vi "动力和环境监控系统首页.vi"() -> ()   [LabVIEW 2016, in "环境动力监测库.lvlib"]
panel:
  out "网络状态":bool
  out "安防模块":T1
  out "暖通模块":T2
  out "供电模块":T3 {"蓄电池"."电量" format="%.0f %"; "蓄电池"."电池电量:" scale=0.0..100.0; "UPS"."电量" format="%.0f %"; "UPS"."电池电量:" scale=0.0..100.0}
  # "安防模块"
  # "供电模块"
  # "其他"
  # "暖通模块"
  # "真角"
  # "m/s"
  # "℃"
  # "bars"
  # "℃"
  # "℃"
  # "℃"
  # "V"
  # "V"
  # "V"
  # "V"
  # "V"
  # "A"
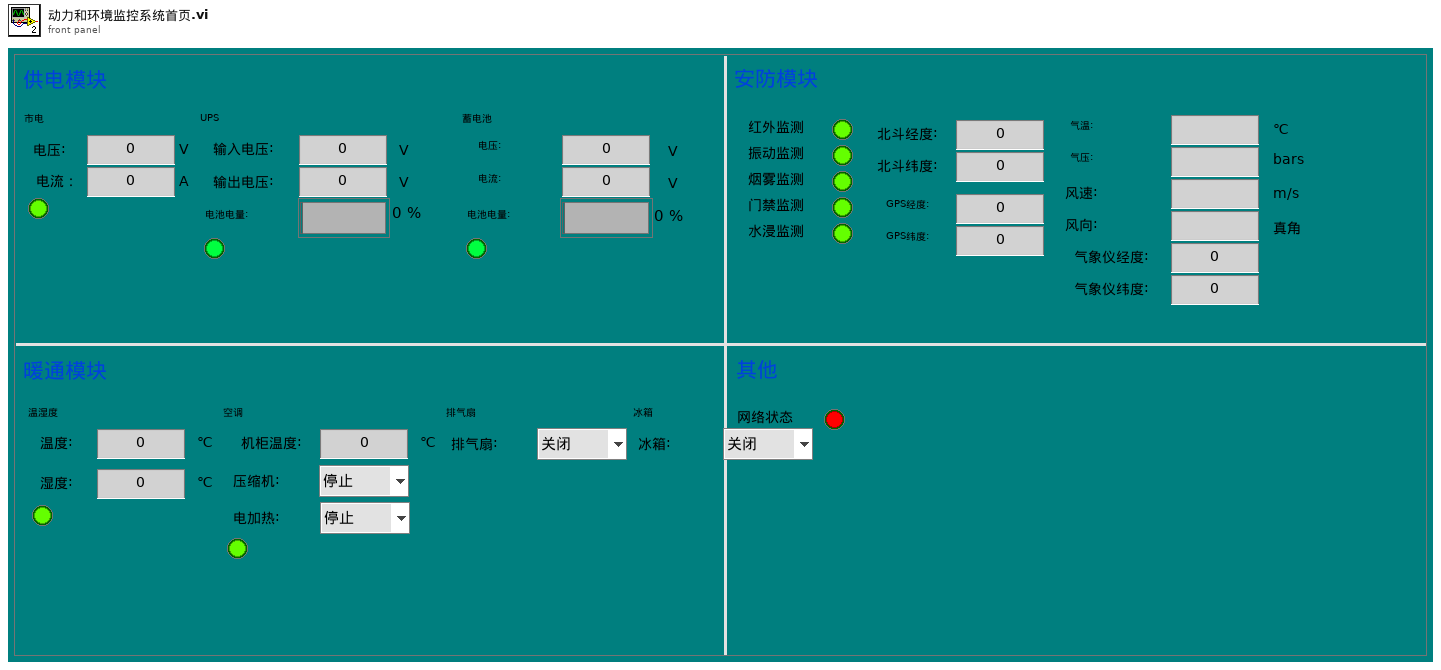
[diagram p1: front panel]
types:
  T1 = cluster{"传感器":cluster{"红外监测":bool, "振动监测":bool, "烟雾监测":bool, "门禁监测":bool, "水浸监测":bool}, "北斗-GPS":cluster{"北斗":cluster{"北斗经度:":sgl, "北斗纬度:":sgl}, "GPS":cluster{"GPS经度: ":sgl, "GPS纬度: ":sgl}}, "气象仪":cluster{"气温: ":sgl, "气压: ":sgl, "风速:":sgl, "风向:":sgl, "气象仪经度: ":sgl, "气象仪纬度: ":sgl}}
  T2 = cluster{"温湿度":cluster{"温度:":sgl, "状态":bool, "湿度:":sgl}, "空调":cluster{"机柜温度:":sgl, "状态":bool, "压缩机:":enum16{"停止", "运行"}, "电加热:":enum16{"停止", "运行"}}, "排气扇":cluster{"排气扇:":enum16{"关闭", "打开"}}, "冰箱":cluster{"冰箱:":enum16{"关闭", "打开"}}}
  T3 = cluster{"市电":cluster{"电压:":u16, "电流：":dbl, "状态":bool}, "UPS":cluster{"输入电压:":sgl, "输出电压:":sgl, "电池电量:":u8, "电量":u16, "状态 2":bool}, "蓄电池":cluster{"电压:":sgl, "电流:":sgl, "电池电量:":u8, "电量":u16, "状态":bool}}
  T4 = cluster{"市电":cluster{"电压:":u16, "电流：":dbl, "状态":bool}, "UPS":cluster{"输入电压:":sgl, "输出电压:":sgl, "电池电量:":u8, "电量":u16, "状态":bool}, "蓄电池":cluster{"电压:":sgl, "电流:":sgl, "电池电量:":u8, "电量":u16, "状态":bool}}
  T5 = cluster{"市电监测":bool, "用水量监测":bool, "烟雾监测":bool, "温度湿度":bool, "振动监测":bool, "红外入侵监测":bool, "漏水监测":bool, "门禁开关监测":bool, "视频监测":bool, "UPS监测":bool, "空调监测":bool, "冰箱监测":bool, "排气扇监测":bool, "蓄电池监测":bool, "GPS监测":bool, "北斗监测":bool, "气象监测":bool}
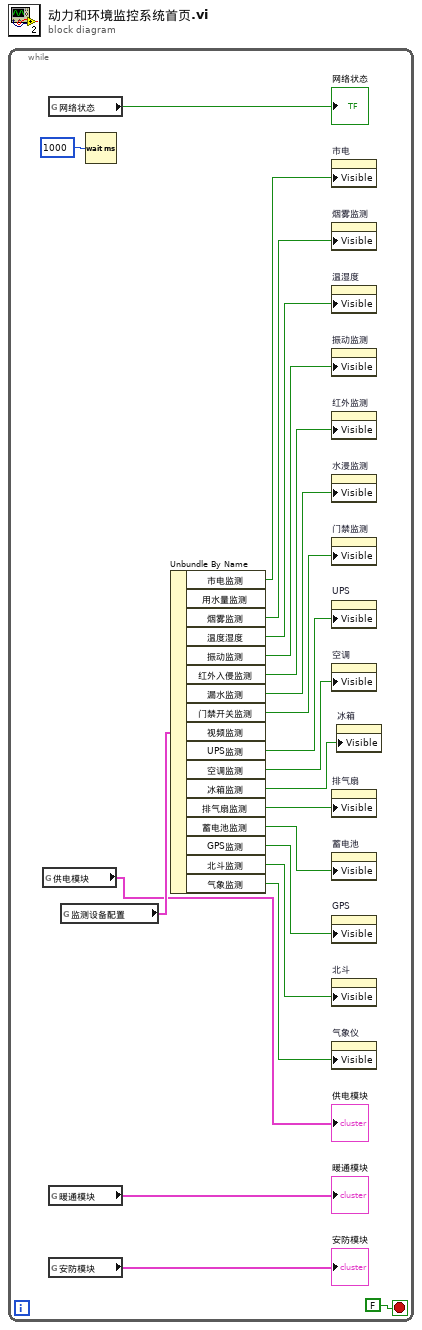
[diagram p0: block diagram]
diagram:
  n1 = while {
    stop <- FALSE stop-if-true
    n2 = global read "内部交互全局变量.vi" "供电模块"() -> (→"供电模块":T4)
    n3 = global read "内部交互全局变量.vi" "网络状态"() -> (→"网络状态":bool)
    n4 = global read "内部交互全局变量.vi" "暖通模块"() -> (→"暖通模块":T2)
    n5 = global read "内部交互全局变量.vi" "安防模块"() -> (→"安防模块":T1)
    n6 = global read "断电保存全局变量.vi" "监测设备配置"() -> (w22:T5)
    n7 = Wait (ms)(milliseconds to wait=u32 1000 ("等待时间（毫秒）")) -> ()  [unwired: 1 out]
    n8 = Unbundle By Name(w22) -> ("市电监测"=w10:bool, "烟雾监测"=w18:bool, "温度湿度"=w9:bool, "振动监测"=w17:bool, "红外入侵监测"=w16:bool, "漏水监测"=w15:bool, "门禁开关监测"=w14:bool, "UPS监测"=w8:bool, "空调监测"=w5:bool, "冰箱监测"=w1:bool, "排气扇监测"=w6:bool, "蓄电池监测"=w7:bool, "GPS监测"=w4:bool, "北斗监测"=w3:bool, "气象监测"=w2:bool)  [unwired: 2 out]
    n9 = property on="市电" class="Clust (严格)"("Visible"=w10) -> ()  [unwired: 2 in, 2 out]
    n10 = property on="烟雾监测" class="Bool (严格)"("Visible"=w18) -> ()  [unwired: 2 in, 2 out]
    n11 = property on="温湿度" class="Clust (严格)"("Visible"=w9) -> ()  [unwired: 2 in, 2 out]
    n12 = property on="振动监测" class="Bool (严格)"("Visible"=w17) -> ()  [unwired: 2 in, 2 out]
    n13 = property on="红外监测" class="Bool (严格)"("Visible"=w16) -> ()  [unwired: 2 in, 2 out]
    n14 = property on="水浸监测" class="Bool (严格)"("Visible"=w15) -> ()  [unwired: 2 in, 2 out]
    n15 = property on="门禁监测" class="Bool (严格)"("Visible"=w14) -> ()  [unwired: 2 in, 2 out]
    n16 = property on="UPS" class="Clust (严格)"("Visible"=w8) -> ()  [unwired: 2 in, 2 out]
    n17 = property on="空调" class="Clust (严格)"("Visible"=w5) -> ()  [unwired: 2 in, 2 out]
    n18 = property on="排气扇" class="Clust (严格)"("Visible"=w6) -> ()  [unwired: 2 in, 2 out]
    n19 = property on="蓄电池" class="Clust (严格)"("Visible"=w7) -> ()  [unwired: 2 in, 2 out]
    n20 = property on="GPS" class="Clust (严格)"("Visible"=w4) -> ()  [unwired: 2 in, 2 out]
    n21 = property on="北斗" class="Clust (严格)"("Visible"=w3) -> ()  [unwired: 2 in, 2 out]
    n22 = property on="气象仪" class="Clust (严格)"("Visible"=w2) -> ()  [unwired: 2 in, 2 out]
    n23 = property on="冰箱" class="Clust (严格)"("Visible"=w1) -> ()  [unwired: 2 in, 2 out]
  }
